vi "2.2 малый экран.vi"() -> (11 "Image":T1(plugin-control))   [LabVIEW 2011]
panel:
  in  "Положение толкателя":dbl(slide) scale=0.0..100.0
  in  "Переменная зазора":dbl
  in  "ток барабана 1":dbl
  in  "Скорость вращения":dbl
  in  "Температура камеры":dbl
  out "Температура\nподшипника":string
  in  "Температура ролика":dbl
  out "Температура ролика":string
  out "Давление в камере":string
  in  "Давление в камере":dbl
  out "Частота вращения заготовки (1000/мин)":string
  out "PV  зазор (мм)":string
  in  "stop":bool
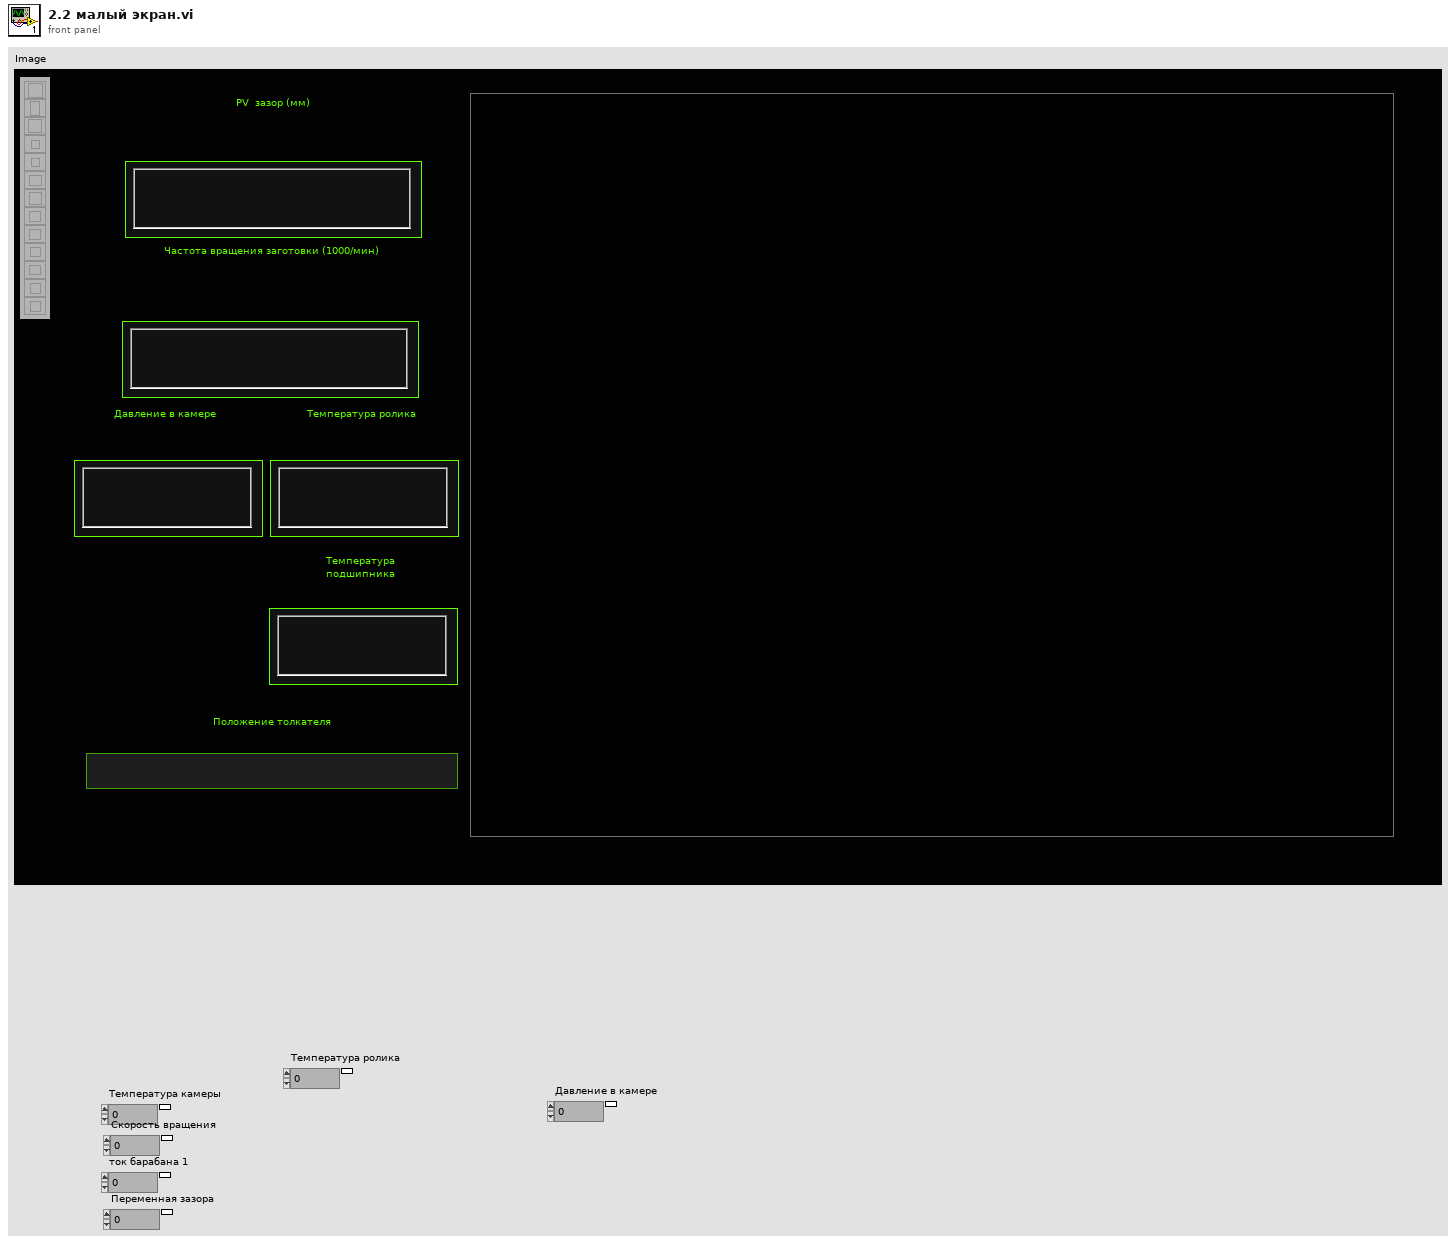
[diagram p1: front panel]
types:
  T1 = typedef "IMAQ Image.ctl" = refnum<image>
  T2 = typedef "Image Type" = u32
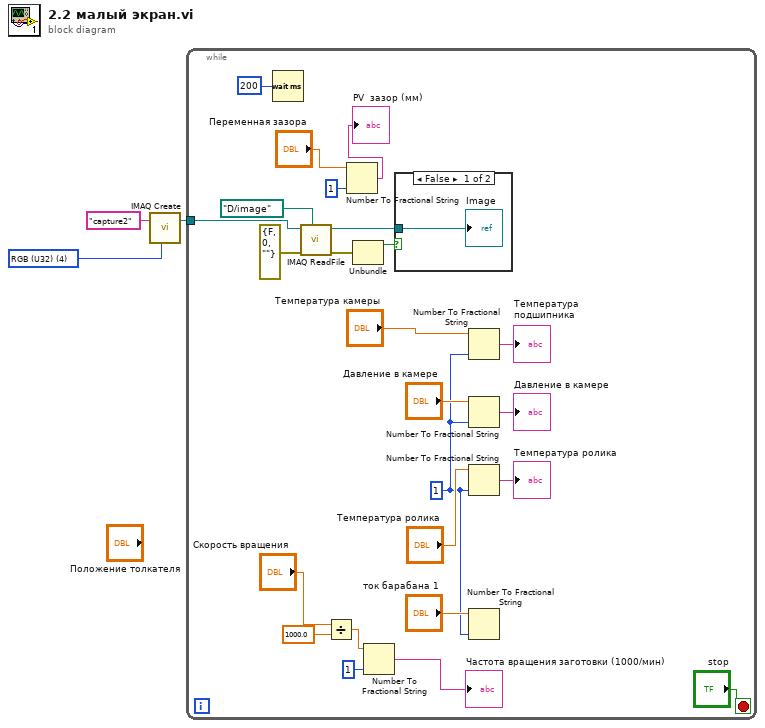
[diagram p0: block diagram]
diagram:
  w2 = T2 4 items=["Grayscale (U8)", "Grayscale (I16)", "Grayscale (SGL)", "Complex (CSG)", "RGB (U32)", "HSL (U32)", "RGB (U64)", "Grayscale (U16)"] ("Image Type")
  n1 = call "IMAQ Create"("Image Name"="capture2", "Image Type"=w2) -> ("New Image"=w1:T1)  [unwired: 3 in, 1 out]
  n2 = while {
    tunnel: w1 -> [w21]
    stop <- "stop" stop-if-true
    w13 = i16 1 ("precision (6)")
    n3 = Wait (ms)(milliseconds to wait=u32 200 ("millisecond multiple")) -> ()  [unwired: 1 out]
    n4 = call "IMAQ ReadFile"("File Path"=path "D:/image", "error in (no error)"=errorcluster {"status"=FALSE, "code"=0, "source"=""}, "Image"=w21) -> ("error out"=w22:errorcluster, "Image Out"=w25:T1)  [unwired: 4 in, 3 out]
    n5 = Divide(x="Скорость вращения", y=1000.0) -> (x/y=w9:dbl)
    n6 = Number To Fractional String(number="Переменная зазора", precision (6)=i16 1) -> (F-format string=→"PV  зазор (мм)":string)  [unwired: 2 in]
    n7 = Unbundle(w22) -> ("status"=w20:bool)  [unwired: 2 out]
    n8 = Number To Fractional String(number=w9, precision (6)=i16 1) -> (F-format string=→"Частота вращения заготовки (1000/мин)":string)  [unwired: 2 in]
    n9 = case shown="False" w20 {
      tunnel: w25 -> [w28 _]
      frame False {
        "Image" <- w28
      }
      frame True {
      }
    }
    n10 = Number To Fractional String(number="Температура камеры", precision (6)=w13) -> (F-format string=→"Температура\nподшипника":string)  [unwired: 2 in]
    n11 = Number To Fractional String(number="Давление в камере", precision (6)=w13) -> (F-format string=→"Давление в камере":string)  [unwired: 2 in]
    n12 = Number To Fractional String(number="Температура ролика", precision (6)=w13) -> (F-format string=→"Температура ролика":string)  [unwired: 2 in]
    n13 = Number To Fractional String(number="ток барабана 1", precision (6)=w13) -> ()  [unwired: 2 in, 1 out]
  }
